vi "DisableAllControlled.vi"(6 "Cell Position":T1, 8 "error in (no error)":errorcluster, 9 "Col Array Ref in":refnum<vi>, 10 "Table CtlRef in":refnum<vi>, 11 "MenuDisableCol in":refnum<class "MenuDisableCol.lvclass">) -> (0 "error out":errorcluster, 1 "Col Array Ref out":refnum<vi>, 2 "Table CtlRef out":refnum<vi>, 3 "MenuDisableCol out":refnum<class "MenuDisableCol.lvclass">)   [LabVIEW 2013, in "MenuDisableCol.lvclass"]
uses:
  MenuDisableCol.lvclass
  <vilib>/Utility/miscctls.llb/LVRowAndColumnTypeDef.ctl
  MenuDisableCol.lvclass/MenuDisableCol.ctl
  Column/Column.lvclass
  Globals/DisabledColorGlobal.vi
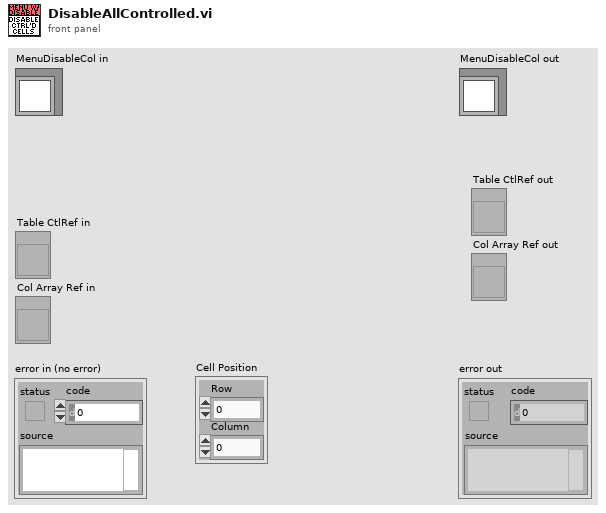
[diagram p1: front panel]
types:
  T1 = typedef "LVRowAndColumnTypeDef.ctl" = cluster{"Row":i32, "Column":i32}
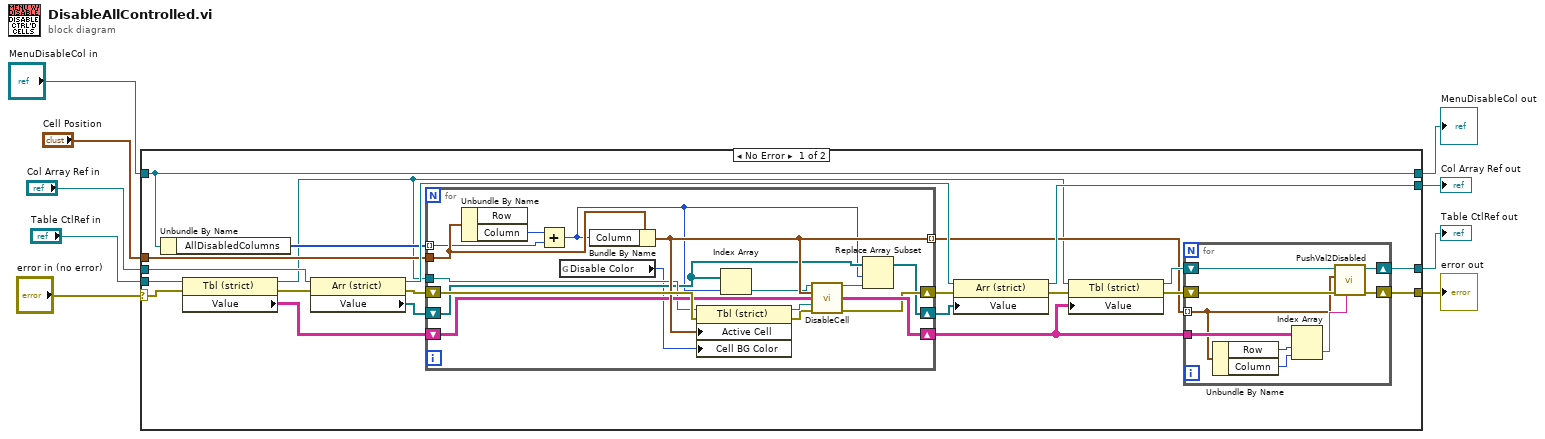
[diagram p0: block diagram]
diagram:
  n1 = case shown="No Error" "error in (no error)" {
    selector: "error in (no error)" -> [w11 w61]
    tunnel: [w17 w61] -> w8
    tunnel: [w10 w60] -> w6
    tunnel: "MenuDisableCol in" -> [w10 w60]
    tunnel: "Table CtlRef in" -> [w23 w59]
    tunnel: [w18 w59] -> w4
    tunnel: "Col Array Ref in" -> [w31 w58]
    tunnel: [w28 w58] -> w2
    tunnel: "Cell Position" -> [w13 _]
    frame No Error {
      n2 = Unbundle By Name(w10) -> ("AllDisabledColumns"=w20:i32[])
      n3 = property class="Tbl (strict)"(reference=w23, error in=w11) -> (reference out=w12:refnum<vi>, error out=w21:errorcluster, "Value"=w22:string[][])
      n4 = property class="Arr (strict)"(reference=w31, error in=w21) -> (reference out=w27:refnum<vi>, error out=w29:errorcluster, "Value"=w30:refnum<class "Column.lvclass">[])
      n5 = for {
        tunnel: w20 -> [w55] mode=indexing
        shift-right: [w45] -> w26
        shift-left: w30 -> [w46]
        shift-right: [w51] -> w25
        shift-left: w29 -> [w54]
        shift-right: [w52] -> w15
        shift-left: w22 -> [w50]
        tunnel: [w53] -> w14 mode=indexing
        tunnel: w13 -> [w57]
        tunnel: w12 -> [w49]
        n6 = Unbundle By Name(w57) -> ("Column"=w56:i32)  [unwired: 1 out]
        n7 = Add(x=w56, y=w55) -> (x+y=w44:i32)
        n8 = global read "DisabledColorGlobal.vi" "Disable Color"() -> (w41:u32)
        n9 = Bundle By Name(cluster=w57, "Column"=w44) -> (w53:T1)
        n10 = property class="Tbl (strict)"(reference=w49, error in=w54, "Active Cell"=w53, "Cell BG Color"=w41) -> (reference out=w43:refnum<vi>, error out=w42:errorcluster)
        n11 = Index Array(array=w46, index=w44) -> (element=w48:refnum<class "Column.lvclass">)
        n12 = call-dynamic "DisableCell.vi"("Column in"=w48, "Cell Position"=w53, "Table Data in"=w50, "Table CtlRef In"=w43, "error in (no error)"=w42) -> ("Column out"=w47:refnum<class "Column.lvclass">, "Table Data out"=w52:string[][], "error out"=w51:errorcluster)  [unwired: 7 in, 1 out]
        n13 = Replace Array Subset(array=w46, new element=w47, index=w44) -> (w45:refnum<class "Column.lvclass">[])
      }
      n14 = property class="Arr (strict)"(reference=w27, error in=w25, "Value"=w26) -> (reference out=w28:refnum<vi>, error out=w24:errorcluster)
      n15 = property class="Tbl (strict)"(reference=w12, error in=w24, "Value"=w15) -> (reference out=w19:refnum<vi>, error out=w16:errorcluster)
      n16 = for {
        shift-right: [w39] -> w18
        shift-left: w19 -> [w40]
        shift-right: [w38] -> w17
        shift-left: w16 -> [w37]
        tunnel: w15 -> [w36]
        tunnel: w14 -> [w32] mode=indexing
        n17 = Unbundle By Name(w32) -> ("Row"=w34:i32, "Column"=w33:i32)
        n18 = Index Array(array=w36, index (row)=w34, index (col)=w33) -> (element=w35:string)
        n19 = call "PushVal2Disabled.vi"("Value"=w35, "error in (no error)"=w37, "Cell Position"=w32, "Table CtlRef In"=w40) -> ("error out"=w38:errorcluster, "Table CtlRef Out"=w39:refnum<vi>)  [unwired: 5 in, 1 out]
      }
    }
    frame Error {
    }
  }
  "error out" <- w8
  "MenuDisableCol out" <- w6
  "Table CtlRef out" <- w4
  "Col Array Ref out" <- w2
